vi "FPGAPowerMeasurement3.vi"() -> ()   [LabVIEW 2009]
uses:
  <vilib>/Waveform/DWDTOps.llb/Digital Pattern Generator (Toggle).vi
panel:
  out "Voltage":dynamicdata(graph)
  out "Power":dynamicdata(graph)
  out "Average Power":dbl
  out "Average Voltage":dbl
  out "Average Current":dbl
  out "Current":dynamicdata(graph)
  in  "stop":bool
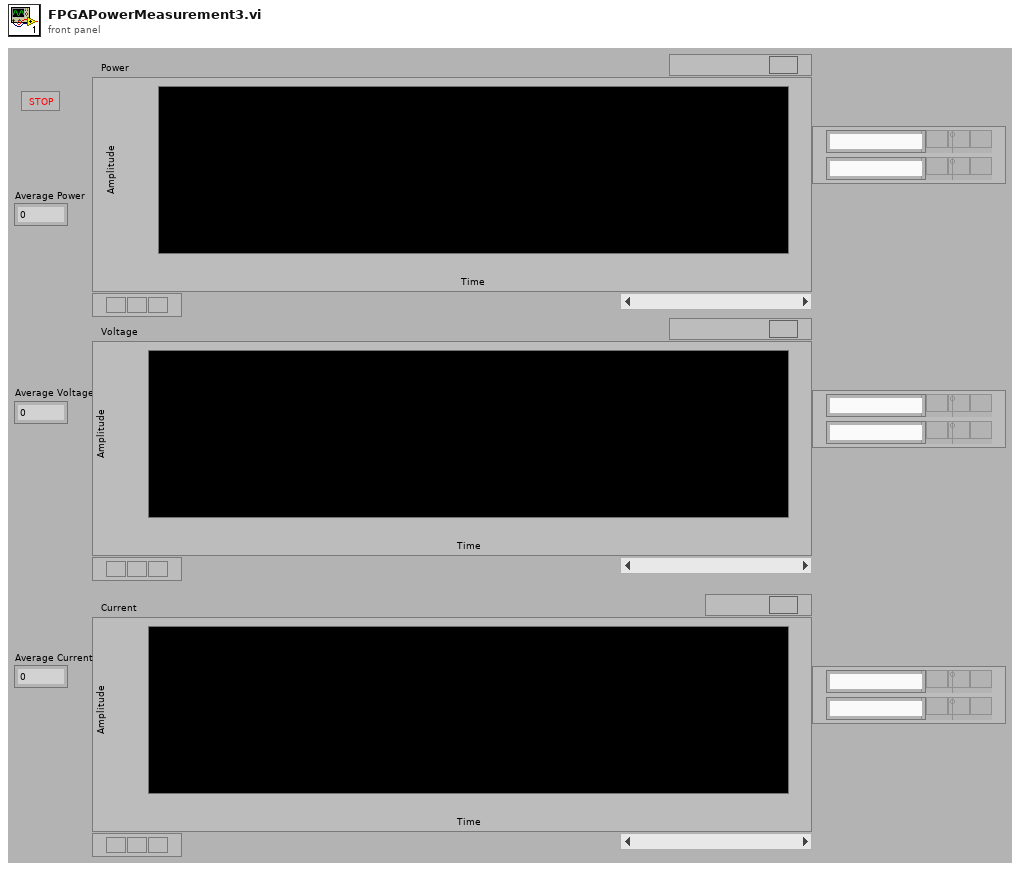
[diagram p1: front panel]
types:
  T1 = typedef "LVTextColorsTypeDef.ctl" = cluster{"Text Color":u32, "Background Color":u32}
  T2 = typedef "LVRangeTypeDef.ctl" = cluster{"Minimum":dbl, "Maximum":dbl, "Increment":dbl, "Minor Increment":dbl, "Start":dbl}
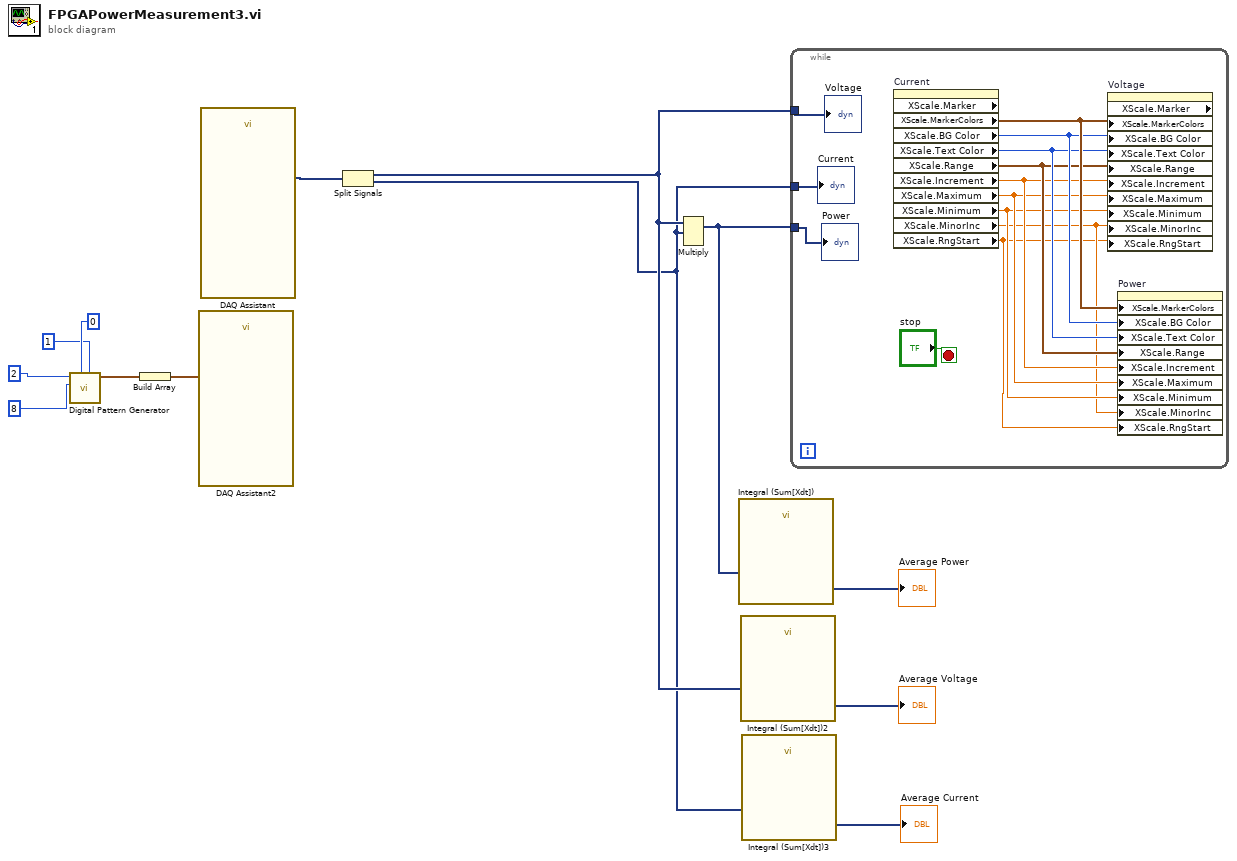
[diagram p0: block diagram]
diagram:
  n1 = call-poly <vilib>:"Digital Pattern Generator.vi"("value 2"=1, "value 1"=0, "number of signals"=8, "number of samples"=2) -> ("digital waveform"=w7:digitalwaveform)  [unwired: 6 in, 1 out]
  n2 = Build Array(w7) -> (w8:digitalwaveform[])
  n3 = call "DAQ Assistant2"("data"=w8) -> ()  [unwired: 17 in, 2 out]
  n4 = call "DAQ Assistant"() -> ("data"=w9:dynamicdata)  [unwired: 17 in, 2 out]
  n5 = Split Signals(w9) -> (w2:dynamicdata, w1:dynamicdata)  [unwired: 2 in]
  n6 = Multiply(1:w1, 2:w2) -> (0:w13:dynamicdata)  [unwired: 1 in, 1 out]
  n7 = call "Integral (Sum[Xdt])"("Signals"=w13) -> ("Result"=→"Average Power":dynamicdata)  [unwired: 5 in, 1 out]
  n8 = call "Integral (Sum[Xdt])2"("Signals"=w2) -> ("Result"=→"Average Voltage":dynamicdata)  [unwired: 5 in, 1 out]
  n9 = call "Integral (Sum[Xdt])3"("Signals"=w1) -> ("Result"=→"Average Current":dynamicdata)  [unwired: 5 in, 1 out]
  n10 = while {
    tunnel: w2 -> [w24]
    tunnel: w1 -> [w25]
    tunnel: w13 -> [w23]
    stop <- "stop" stop-if-true
    n11 = property on="Current" class="WFGraph (strict)" props=["XScale", "Marker", "XScale", "MarkerColors", "XScale", "BG Color", "XScale", "Text Color", "XScale", "Range", "XScale", "Increment", "XScale", "Maximum", "XScale", "Minimum", "XScale", "MinorInc", "XScale", "RngStart"]() -> ("XScale.MarkerColors"=w22:T1, "XScale.BG Color"=w21:u32, "XScale.Text Color"=w20:u32, "XScale.Range"=w19:T2, "XScale.Increment"=w18:dbl, "XScale.Maximum"=w17:dbl, "XScale.Minimum"=w16:dbl, "XScale.MinorInc"=w15:dbl, "XScale.RngStart"=w14:dbl)  [unwired: 2 in, 3 out]
    n12 = property on="Voltage" class="WFGraph (strict)" props=["XScale", "Marker", "XScale", "MarkerColors", "XScale", "BG Color", "XScale", "Text Color", "XScale", "Range", "XScale", "Increment", "XScale", "Maximum", "XScale", "Minimum", "XScale", "MinorInc", "XScale", "RngStart"]("XScale.MarkerColors"=w22, "XScale.BG Color"=w21, "XScale.Text Color"=w20, "XScale.Range"=w19, "XScale.Increment"=w18, "XScale.Maximum"=w17, "XScale.Minimum"=w16, "XScale.MinorInc"=w15, "XScale.RngStart"=w14) -> ()  [unwired: 2 in, 3 out]
    n13 = property on="Power" class="WFGraph (strict)"("XScale.MarkerColors"=w22, "XScale.BG Color"=w21, "XScale.Text Color"=w20, "XScale.Range"=w19, "XScale.Increment"=w18, "XScale.Maximum"=w17, "XScale.Minimum"=w16, "XScale.MinorInc"=w15, "XScale.RngStart"=w14) -> ()  [unwired: 2 in, 2 out]
    "Current" <- w25
    "Power" <- w23
    "Voltage" <- w24
  }
